vi "AddScreenshots.vi"(8 "error in (no error)":errorcluster, 9 "Screenshot Type":T3, 10 "Screenshot Paths":path[](array[path]), 11 "VI Screenshots In":T1) -> (0 "error out":errorcluster, 3 "VI Screenshots Out":T1)   [LabVIEW 2020, in "VIDiffScreenshots.lvlib"]
uses:
  VIDiffScreenshots.lvlib
  VIScreenshots.ctl
  ScreenshotInfo.ctl
  Screenshot Type.ctl
  Utilities/FilePaths.ctl
  Utilities/VIDiffUtilities.lvlib
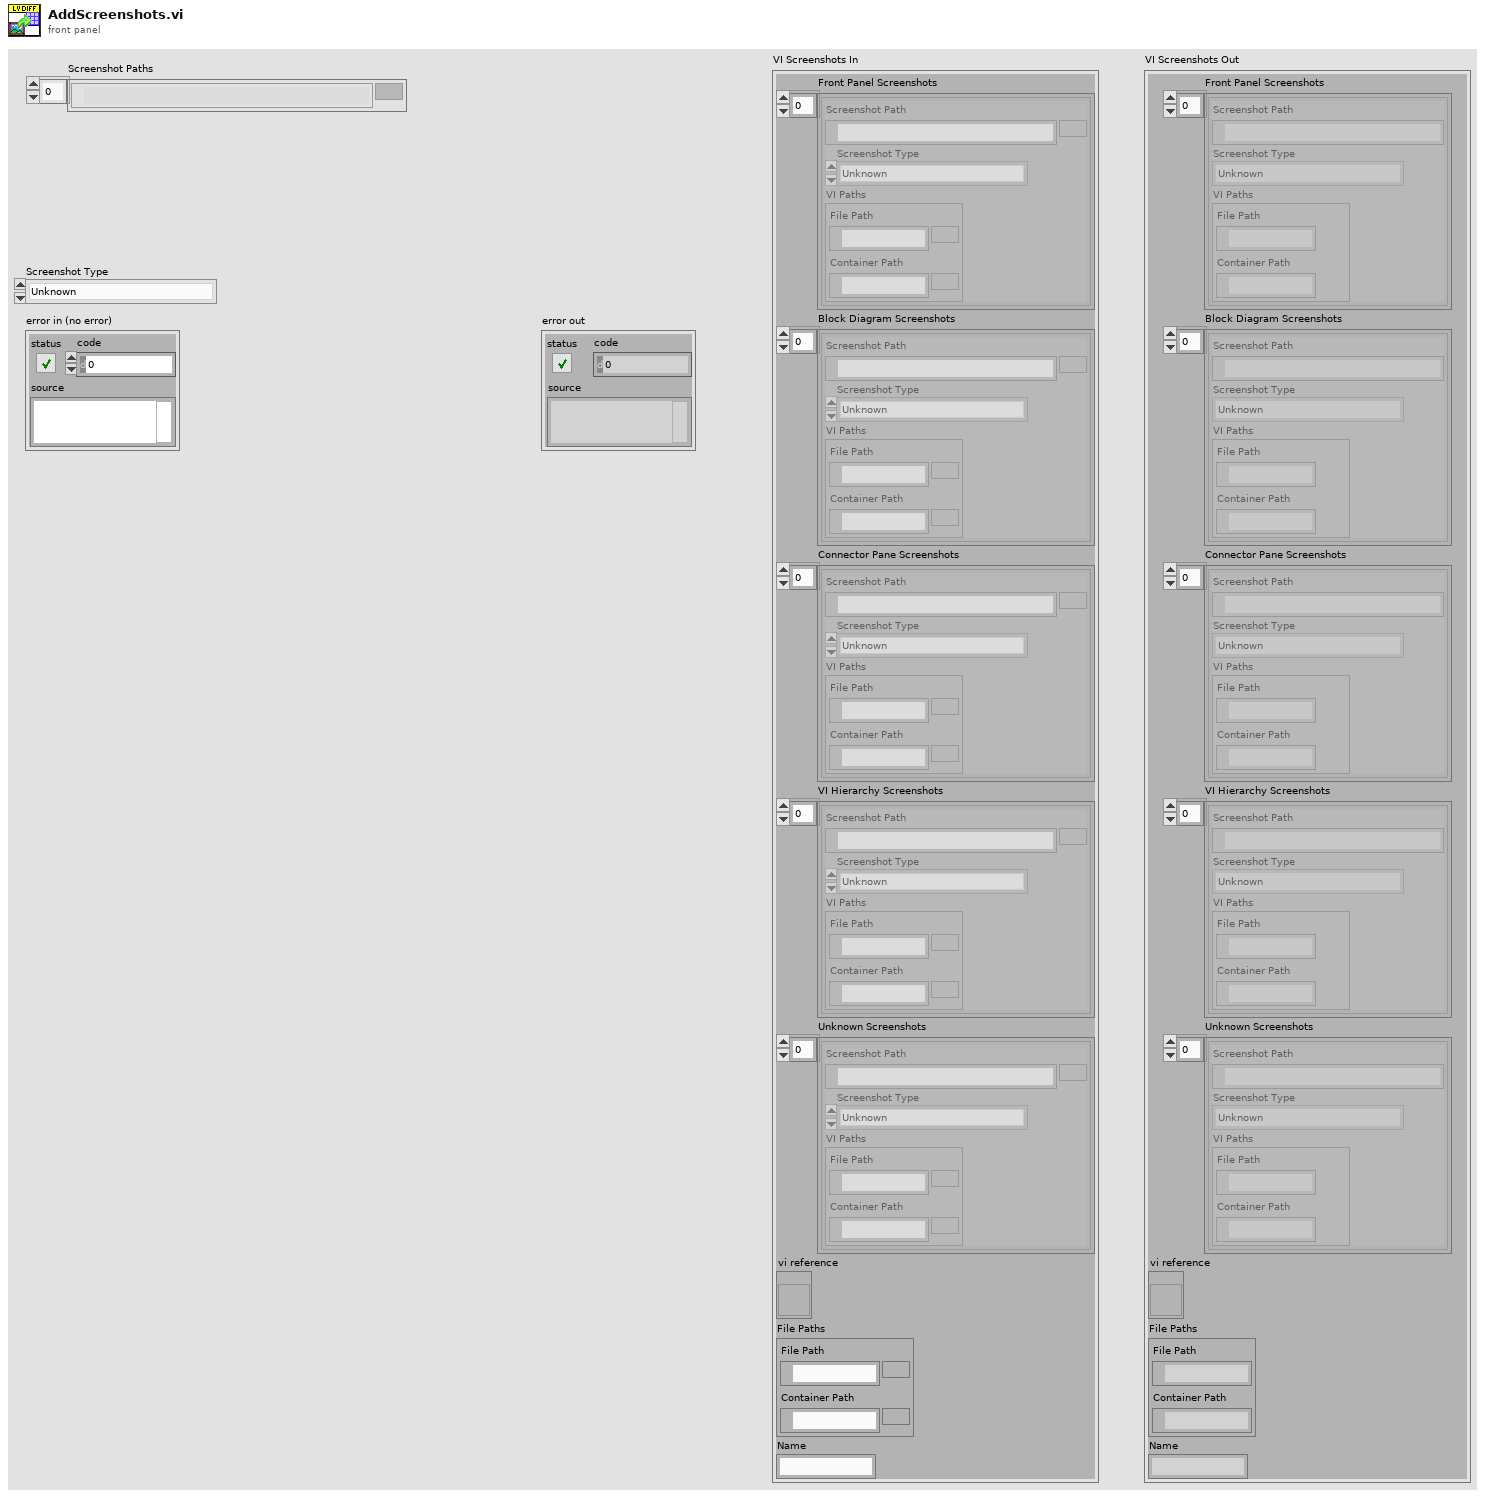
[diagram p1: front panel]
types:
  T1 = typedef "VIDiffScreenshots.lvlib/VIScreenshots.ctl" = cluster{"Front Panel Screenshots":T2[], "Block Diagram Screenshots":T2[], "Connector Pane Screenshots":T2[], "VI Hierarchy Screenshots":T2[], "Unknown Screenshots":T2[], "vi reference":refnum<vi>, "File Paths":cluster{"File Path":path, "Container Path":path}, "Name":string}
  T2 = typedef "VIDiffScreenshots.lvlib/ScreenshotInfo.ctl" = cluster{"Screenshot Path":path, "Screenshot Type":T3, "VI Paths":T4}
  T3 = typedef "VIDiffScreenshots.lvlib/Screenshot Type.ctl" = enum16{"Unknown", "Front Panel", "Connector Pane", "Block Diagram", "VI Hierarchy"}
  T4 = typedef "VIDiffUtilities.lvlib/FilePaths.ctl" = cluster{"File Path":path, "Container Path":path}
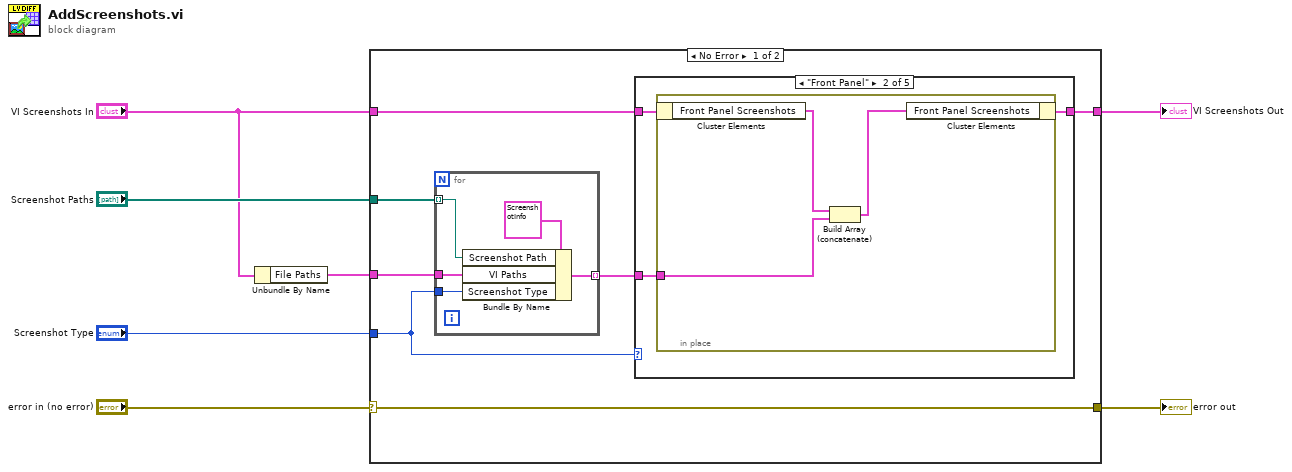
[diagram p0: block diagram]
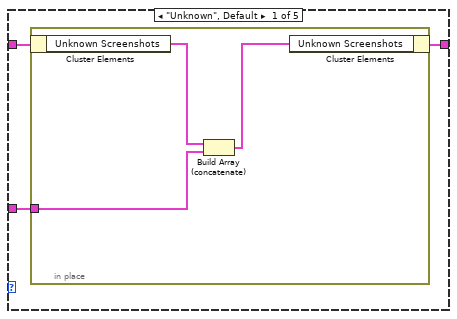
[diagram p2: hidden frame]
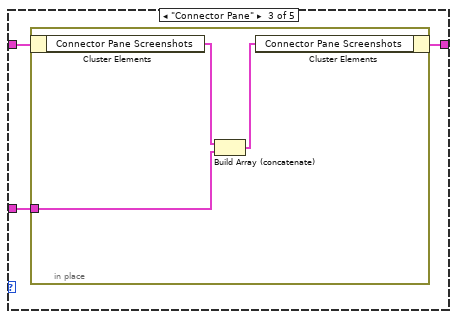
[diagram p3: hidden frame]
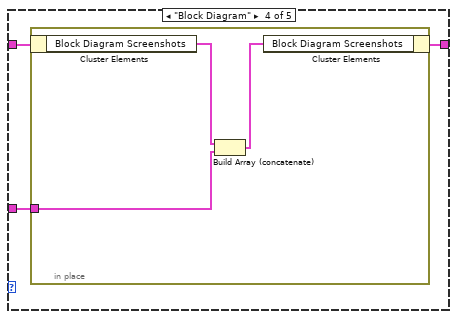
[diagram p4: hidden frame]
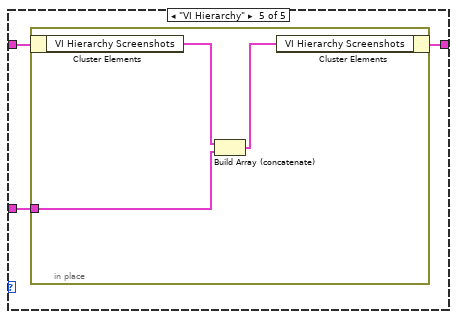
[diagram p5: hidden frame]
diagram:
  n1 = Unbundle By Name("VI Screenshots In") -> ("File Paths"=w1:cluster{"File Path":path, "Container Path":path})
  n2 = case shown="No Error" "error in (no error)" {
    selector: "error in (no error)" -> [w14 w51]
    tunnel: [w14 w51] -> w6
    tunnel: "VI Screenshots In" -> [w9 w50]
    tunnel: "Screenshot Type" -> [w10 _]
    tunnel: [w8 w50] -> w4
    tunnel: "Screenshot Paths" -> [w13 _]
    tunnel: w1 -> [w12 _]
    frame No Error {
      n3 = for {
        tunnel: w13 -> [w48] mode=indexing
        tunnel: w10 -> [w47]
        tunnel: w12 -> [w46]
        tunnel: [w45] -> w11 mode=indexing
        n4 = Bundle By Name(cluster=T2 {"Screenshot Path"=path "", "Screenshot Type"=enum."Unknown", "VI Paths"={"File Path"=path "", "Container Path"=path ""}} ("Screenshot Info"), "Screenshot Path"=w48, "VI Paths"=w46, "Screenshot Type"=w47) -> (w45:T2)
      }
      n5 = case shown="\"Front Panel\"" w10 {
        tunnel: w11 -> [w17 w23 w29 w35 w41]
        tunnel: w9 -> [w16 w22 w28 w34 w40]
        tunnel: [w15 w21 w27 w33 w39] -> w8
        frame "Unknown", Default {
          n6 = in-place {
            in-place-border: w17 -> [w20]
            n7 = in-place-cluster #1(w16) -> ("Unknown Screenshots"=w19:T2[])
            n8 = Build Array (concatenate)(w19, w20) -> (w18:T2[])
            n9 = in-place-cluster #1("Unknown Screenshots"=w18) -> (w15:T1)
          }
        }
        frame "Front Panel" {
          n10 = in-place {
            in-place-border: w23 -> [w26]
            n11 = in-place-cluster #2(w22) -> ("Front Panel Screenshots"=w25:T2[])
            n12 = Build Array (concatenate)(w25, w26) -> (w24:T2[])
            n13 = in-place-cluster #2("Front Panel Screenshots"=w24) -> (w21:T1)
          }
        }
        frame "Connector Pane" {
          n14 = in-place {
            in-place-border: w29 -> [w32]
            n15 = in-place-cluster #3(w28) -> ("Connector Pane Screenshots"=w31:T2[])
            n16 = Build Array (concatenate)(w31, w32) -> (w30:T2[])
            n17 = in-place-cluster #3("Connector Pane Screenshots"=w30) -> (w27:T1)
          }
        }
        frame "Block Diagram" {
          n18 = in-place {
            in-place-border: w35 -> [w38]
            n19 = in-place-cluster #4(w34) -> ("Block Diagram Screenshots"=w37:T2[])
            n20 = Build Array (concatenate)(w37, w38) -> (w36:T2[])
            n21 = in-place-cluster #4("Block Diagram Screenshots"=w36) -> (w33:T1)
          }
        }
        frame "VI Hierarchy" {
          n22 = in-place {
            in-place-border: w41 -> [w44]
            n23 = in-place-cluster #5(w40) -> ("VI Hierarchy Screenshots"=w43:T2[])
            n24 = Build Array (concatenate)(w43, w44) -> (w42:T2[])
            n25 = in-place-cluster #5("VI Hierarchy Screenshots"=w42) -> (w39:T1)
          }
        }
      }
    }
    frame Error {
    }
  }
  "error out" <- w6
  "VI Screenshots Out" <- w4
